vi "Write Parent State.vi"(8 "error in (no error)":errorcluster, 10 "Parent State":refnum<class "State.lvclass">, 11 "Nested State in":refnum<class "Nested State.lvclass">) -> (0 "error out":errorcluster, 3 "Nested State out":refnum<class "Nested State.lvclass">)   [LabVIEW 2024, in "State.lvlib" / "Nested State.lvclass"]
uses:
  Nested State.lvclass
  State/State.lvclass
  Nested State.lvclass/Nested State.ctl
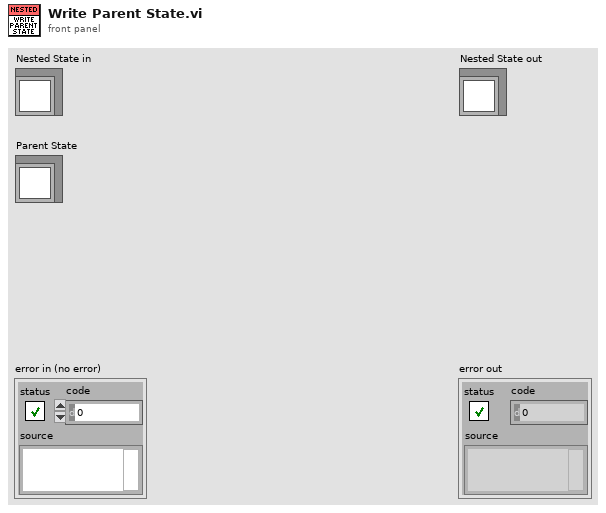
[diagram p1: front panel]
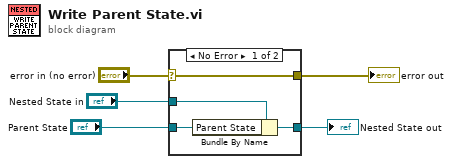
[diagram p0: block diagram]
diagram:
  n1 = case shown="No Error" "error in (no error)" {
    selector: "error in (no error)" -> [w9 w10]
    tunnel: [w9 w10] -> w4
    tunnel: [w7 w11] -> w2
    tunnel: "Nested State in" -> [w8 w11]
    tunnel: "Parent State" -> [w6 _]
    frame No Error {
      n2 = Bundle By Name(cluster=w8, "Parent State"=w6) -> (w7:refnum<class "Nested State.lvclass">)
    }
    frame Error {
    }
  }
  "error out" <- w4
  "Nested State out" <- w2
